vi "Emballage_BDD_Lecture_table_local.vi"(8 "entrée d'erreur (pas d'erreur)":errorcluster) -> (0 "sortie d'erreur":errorcluster, 1 "Dec.Droite 2":string="^LH70,20", 2 "Com Imprimante":string(combo), 3 "Refnum VISA en sortie":refnum<visa-resource-name>, 4 "Imprimante certif":string(combo), 5 "Imprimante Zebra":string(combo), 6 "Result Set":string[][](table) caption="Result Set (from first statement with results)")   [LabVIEW 2020]
uses:
  Modules/FS/60_FS_Controles/60_FS_SetGet.ctl
  <vilib>/drjdpowell/SQLite Library/SQL Connection/Open (path).vi
  <vilib>/drjdpowell/SQLite Library/SQL Connection/Open (string).vi
  <vilib>/AdvancedString/Path To Command Line String.vi
  <vilib>/drjdpowell/SQLite Library/SQL Connection/Connection.lvclass
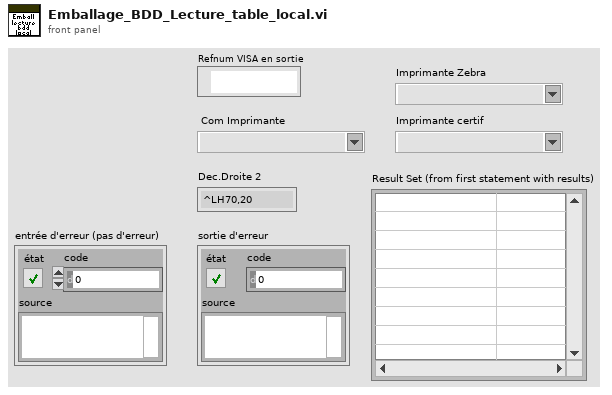
[diagram p1: front panel]
types:
  T1 = typedef "60_FS_SetGet.ctl" = enum16{"set", "get"}
  T2 = typedef "60_FS_CLT_Chemins.ctl" = cluster{"Racine_local":path, "Racine_reseau":path, "Racine_Support_Application":path, "Fichier_Journalisation":path, "Connexion_BDD_VSX":path, "Connexion_BDD_PLZ":path}
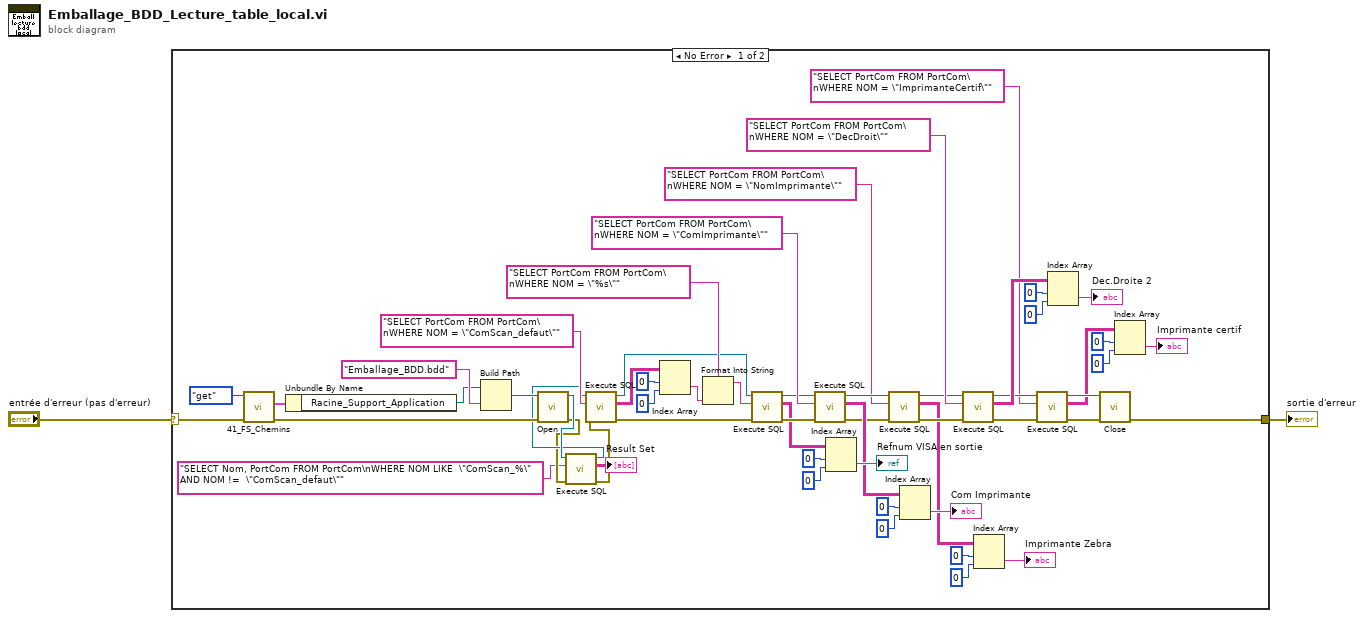
[diagram p0: block diagram]
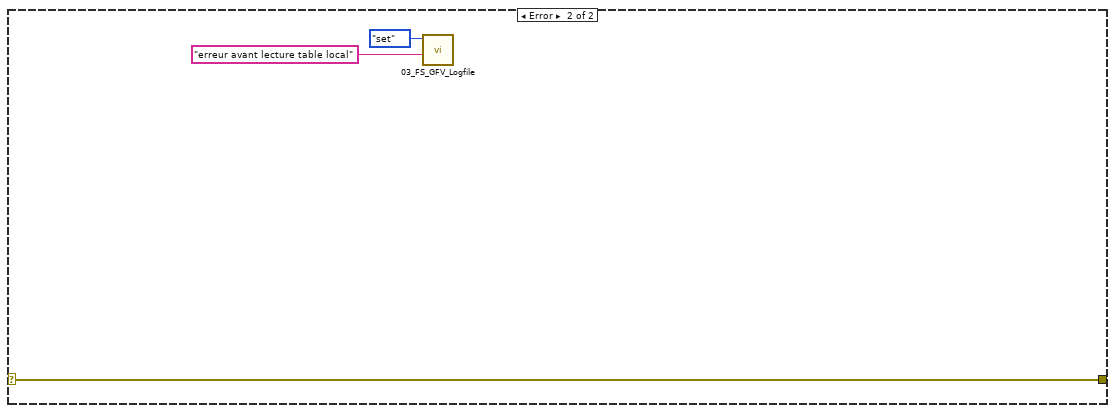
[diagram p2: hidden frame]
diagram:
  n1 = case shown="No Error" "entrée d'erreur (pas d'erreur)" {
    selector: "entrée d'erreur (pas d'erreur)" -> [w36 w62]
    tunnel: [w35 w62] -> w1
    frame No Error {
      n2 = call "41_FS_Chemins.vi"("error in (no error)"=w36, "SetGet"=60_FS_SetGet."get") -> ("error out"=w40:errorcluster, "CLT_Chemins_out"=w38:T2)  [unwired: 8 in]
      n3 = Unbundle By Name(w38) -> ("Racine_Support_Application"=w39:path)
      n4 = Build Path(base path=w39, name or relative path="Emballage_BDD.bdd" ("nom ou chemin relatif")) -> (appended path=w41:path)
      n5 = call-poly <vilib>:"Open.vi"("error in (no error)"=w40, "db file"=w41) -> ("error out"=w6:errorcluster, "SQLite Connection"=w8:refnum<class "Connection.lvclass">)  [unwired: 8 in]
      n6 = call <vilib>:"Execute SQL.vi"("error in (no error)"=w6, "SQL"="SELECT Nom, PortCom FROM PortCom\nWHERE NOM LIKE  \"ComScan_%\" AND NOM !=  \"ComScan_defaut\"", "SQLite Connection in"=w8) -> ("error out"=w5:errorcluster, "Result Set"=→"Result Set":string[][], "SQLite Connection"=w7:refnum<class "Connection.lvclass">)  [unwired: 5 in, 1 out]
      n7 = call <vilib>:"Execute SQL.vi"("error in (no error)"=w5, "SQL"="SELECT PortCom FROM PortCom\nWHERE NOM = \"ComScan_defaut\"", "SQLite Connection in"=w7) -> ("error out"=w14:errorcluster, "Result Set"=w11:string[][], "SQLite Connection"=w15:refnum<class "Connection.lvclass">)  [unwired: 5 in, 1 out]
      n8 = Index Array(array=w11, index (row)=0 ("indice (ligne)"), index (col)=0 ("indice désactivé (col)")) -> (element=w10:string)
      n9 = Format Into String(format string="SELECT PortCom FROM PortCom\nWHERE NOM = \"%s\"" ("SQL"), w10) -> (resulting string=w16:string)  [unwired: 2 in, 1 out]
      n10 = call <vilib>:"Execute SQL.vi"("error in (no error)"=w14, "SQL"=w16, "SQLite Connection in"=w15) -> ("error out"=w48:errorcluster, "Result Set"=w43:string[][], "SQLite Connection"=w47:refnum<class "Connection.lvclass">)  [unwired: 5 in, 1 out]
      n11 = call <vilib>:"Execute SQL.vi"("error in (no error)"=w48, "SQL"="SELECT PortCom FROM PortCom\nWHERE NOM = \"ComImprimante\"", "SQLite Connection in"=w47) -> ("error out"=w25:errorcluster, "Result Set"=w51:string[][], "SQLite Connection"=w22:refnum<class "Connection.lvclass">)  [unwired: 5 in, 1 out]
      n12 = Index Array(array=w43, index (row)=0 ("indice (ligne)"), index (col)=0 ("indice désactivé (col)")) -> (element=→"Refnum VISA en sortie":string)
      n13 = call <vilib>:"Execute SQL.vi"("error in (no error)"=w25, "SQL"="SELECT PortCom FROM PortCom\nWHERE NOM = \"NomImprimante\"", "SQLite Connection in"=w22) -> ("error out"=w24:errorcluster, "Result Set"=w18:string[][], "SQLite Connection"=w23:refnum<class "Connection.lvclass">)  [unwired: 5 in, 1 out]
      n14 = Index Array(array=w51, index (row)=0 ("indice (ligne)"), index (col)=0 ("indice désactivé (col)")) -> (element=→"Com Imprimante":string)
      n15 = call <vilib>:"Execute SQL.vi"("error in (no error)"=w24, "SQL"="SELECT PortCom FROM PortCom\nWHERE NOM = \"DecDroit\"", "SQLite Connection in"=w23) -> ("error out"=w32:errorcluster, "Result Set"=w56:string[][], "SQLite Connection"=w34:refnum<class "Connection.lvclass">)  [unwired: 5 in, 1 out]
      n16 = Index Array(array=w18, index (row)=0 ("indice (ligne)"), index (col)=0 ("indice désactivé (col)")) -> (element=→"Imprimante Zebra":string)
      n17 = call <vilib>:"Execute SQL.vi"("error in (no error)"=w32, "SQL"="SELECT PortCom FROM PortCom\nWHERE NOM = \"ImprimanteCertif\"", "SQLite Connection in"=w34) -> ("error out"=w31:errorcluster, "Result Set"=w26:string[][], "SQLite Connection"=w33:refnum<class "Connection.lvclass">)  [unwired: 5 in, 1 out]
      n18 = Index Array(array=w56, index (row)=0 ("indice (ligne)"), index (col)=0 ("indice désactivé (col)")) -> (element=→"Dec.Droite 2":string)
      n19 = call-dynamic "Close.vi"("error in (no error)"=w31, "SQLite Connection in"=w33) -> ("error out"=w35:errorcluster)  [unwired: 9 in]
      n20 = Index Array(array=w26, index (row)=0 ("indice (ligne)"), index (col)=0 ("indice désactivé (col)")) -> (element=→"Imprimante certif":string)
    }
    frame Error {
      n21 = call "03_FS_GFV_Logfile.vi"("Chaîne"="erreur avant lecture table local", "States"=60_FS_SetGet."set") -> ()  [unwired: 8 in, 2 out]
    }
  }
  "sortie d'erreur" <- w1
